vi "ReadFile.vi"(1 "文件名":string) -> (0 "文件内容":string[](array[string]))   [LabVIEW 2017]
panel:
  in  "error in (no error)":errorcluster caption="错误输入（无错误）"
  out "error out":errorcluster caption="错误输出"
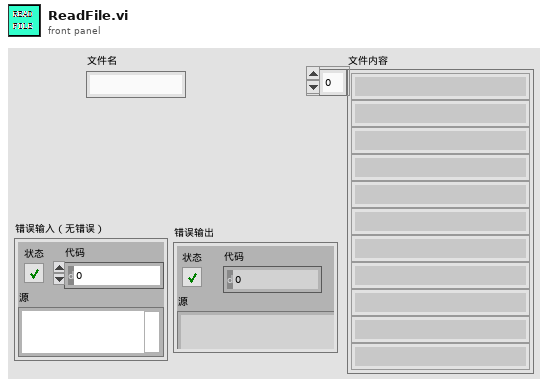
[diagram p1: front panel]
types:
  T1 = enum16{"open", "replace", "create", "open or create", "replace or create", "replace or create with confirmation"}
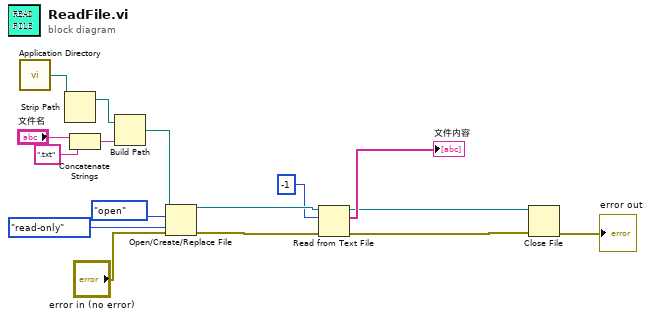
[diagram p0: block diagram]
diagram:
  n1 = call <vilib>:"Application Directory.vi"() -> ("Application Directory"=w16:path)
  n2 = Strip Path(path=w16) -> (stripped path=w15:path)  [unwired: 1 out]
  n3 = Concatenate Strings("文件名", ".txt" ("字符串")) -> (w3:string)
  n4 = Build Path(base path=w15, name or relative path=w3) -> (appended path=w14:path)
  n5 = Open/Create/Replace File(file path (use dialog)=w14, error in="error in (no error)", operation (0:open)=T1."open" ("操作(0:open)"), access (0:read/write)=enum16{"read/write", "read-only", "write-only"}."read-only" ("权限(0:read/write)")) -> (refnum out=w8:refnum<file>, error out=w7:errorcluster)  [unwired: 2 in, 1 out]
  n6 = Read from Text File(file (use dialog)=w8, count=-1 ("计数"), error in=w7) -> (refnum out=w5:refnum<file>, text=→"文件内容":string[], error out=w6:errorcluster)  [unwired: 1 in, 1 out]
  n7 = Close File(refnum=w5, error in=w6) -> (error out=→"error out":errorcluster)  [unwired: 1 out]
